vi "TagDB List Probe.vi"(11 "DB Ref":refnum<k1>) -> (2 "Value String":string, 3 "Boolean":bool)   [LabVIEW 2017]
uses:
  <vilib>/Utility/Data Type/Type Definitions/Data Type.ctl
  <vilib>/Utility/Data Type/Type Definitions/Refnum Type.ctl
  <vilib>/Utility/Data Type/Type Definitions/VI Server Generic Type.ctl
  TagDB/_Support/Change Detector/TagDB dbChanged.vi
  5c30c298-b379-4591-8ff9-b1fc8496978f.vi
  TagDB/_Support/DataAccess/TagDB Ref to DVR.vi
  TagDB/_Support/Error/_[error50000]Invalid DB REF.vi
  TagDB/_Support/Change Detector/TagDB ChangeFlag.vi
  TagDB/_Support/DataAccess/_NameCacher.vi
  TagDB/_Support/Error/_[error50002]Invalid DataType.vi
  TagDB/_Support/URL/TRIM-BOTH-SPACE.vi
  TagDB/_Support/Error/_Build Error Cluster.vi
  TagDB/TagDB.lvlib
  <vilib>/Utility/Data Type/NI_Data Type.lvlib
panel:
  out "Valid?":bool
  out "Name":string
  out "Last Item Change":timestamp format="%<%.3X>T"
  out "Last Data Change":timestamp format="%<%.3X>T"
  in  "Items":i32(listbox)
  out "TagName":string
  out "ValidRef":bool
  out "ClassName":string
  out "Type":T1
  out "Reference Type":T2
  out "VI Server Type":T3
  out "data":variant
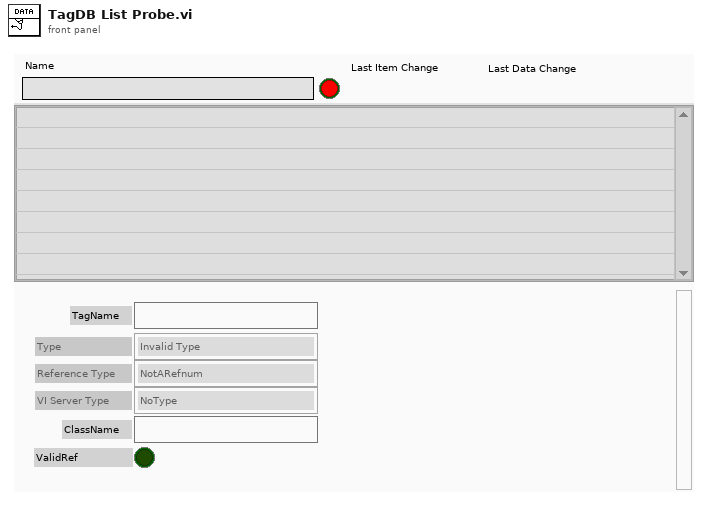
[diagram p1: front panel]
types:
  T1 = typedef "NI_Data Type.lvlib/Data Type.ctl" = enum8{"Invalid Type", "Void", "I8", "I16", "I32", "I64", "U8", "U16", "U32", "U64", "Single Float", "Double Float", "Extended Float", "Single Complex", "Double Complex", "Extended Complex", "Enum U8", "Enum U16", "Enum U32", "Enum U64", "Single Float With Unit", "Double Float With Unit", "Extended Float With Unit", "Single Complex with Unit", "Double Complex with Unit", "Extended Complex with Unit", "Boolean", "String", "Path", "Picture", "Tag", "Array", "Cluster", "Variant", "LV Variant", "Waveform", "Timestamp", "Digital Waveform", "Digital Data", "ExpressData", "Refnum", "External Data", "VI", "Poly VI", "LabVIEW Class Instance", "Fixed Point"}
  T2 = typedef "NI_Data Type.lvlib/Refnum Type.ctl" = enum16{"NotARefnum", "UnknownRefnum", "Generic", "Datalog", "ByteStream", "Device", "Occurence", "TCPNetConnection", "Auto", "Menu", "Imaq", "Hardware", "DataSocket", "Visa", "IVI", "UDPNetConnection", "Notifier", "Queue", "Irda", "EventReg", "DotNet", "UserEvent", "Callback", "UNUSED_EMPTY_POSITION", "BlueToothNetConnection", "LVObjApp", "LVObjVI", "LVObjUnknown", "GenericClass", "UserDefinedRefnumTag", "DataValue", "RT FIFO", "TDMS File"}
  T3 = typedef "NI_Data Type.lvlib/VI Server Generic Type.ctl" = enum16{"NoType", "\tkLVObjApp=0x1", "\tkLVObjVI", "\tkLVObjGeneric", "\tkLVObjDecoration", "\tkLVObjText", "\tkLVObjControl", "\tkLVObjColorBox", "\tkLVObjBoolean", "\tkLVObjRefNum", "\tkLVObjVariant", "\tkLVObjPath", "\tkLVObjListBox", "\tkLVObjTable", "\tkLVObjArray", "\tkLVObjPicture", "\tkLVObjOleContainer", "\tkLVObjNumeric", "\tkLVObjDigital", "\tkLVObjNamedNumeric", "\tkLVObjColorRamp", "\tkLVObjSlide", "\tkLVObjGraphOrChart", "\tkLVObjWaveformChart", "\tkLVObjWaveformGraph", "\tkLVObjIntensityChart", "\tkLVObjIntensityGraph", "\tkLVObjString", "\tkLVObjIOName", "\tkLVObjComboBox", "\tkLVObjCluster", "\tkLVObjPanel", "\tkLVObjKnob", "\tkLVObjNumWithScale", "\tkLVObjRing", "\tkLVObjEnum", "\tkLVObjGObject", "\tkLVObjPlot", "\tkLVObjCursor", "\tkLVObjNumericText", "\tkLVObjScale", "\tkLVObjColorScale", "\tkLVObjGraphScale", "\tkLVObjColorGraphScale", "\tkLVObjTypedRefNum", "\tkLVObjOldKnobScale", "\tkLVObjMCListbox", "\tkLVObjMeasureData", "\tkLVObjDSCTag", "\tkLVObjDAQName", "\tkLVObjVISAName", "\tkLVObjIVIName", "\tkLVObjSlideScale", "\tkLVObjTabControl", "\tkLVObjPage", "\tkLVObjTabArrayTabControl", "\tkLVObjConPane", "\tkLVObjDAQMXName", "\tkLVObjVIRefNum", "\tkLVObjLVObjRefNum", "\tkLVObjAbsTime", "\tkLVObjDigitalTable", "\tkLVObjUnused", "\tkLVObjUnused2", "\tkLVObjSCLControl", "\tkLVObjSubPanel", "\tkLVObjTreeControl", "\tkLVObjGenClassTagRef", "\tkLVObjGenClassRef", "\tkLVObjRotaryColorScale", "\tkLVObjPlugInDDOControl", "\tkLVObjPlugInDDOClassHolder", "\tkLVObjRadClusControl", "\tkLVObjProject", "\tkLVObjProjectItem", "\tkLVObjPane", "\tkLVObjSplitterBar", "\tkLVObjProjectBuildItem", "\tkLVObjPixmap", "\tkLVObjFacadeVI", "\tkLVObjLibrary", "\tkLVObjVariable", "\tkLVObjPropertyBag", "\tkLVObjXYGraph", "\tkLVObjScene", "\tkLVObjUDClassLibrary", "\tkLVObjUDClassClone", "\tkLVObjMethodVI", "\tkLVObjXCtlLibrary", "\tkLVObjXNodeLibrary", "\tkLVObjScroll", "\tkLVObjLVTarget", "\tkLVObjMixedGraph", "\tkLVObjProvider", "\tkLVObjCopyOperation", "\tkLVObjTargetItem", "\tkLVObjProjectItemType", "\tkLVObjCopyItem", "\tkLVObjCopyConflict", "\tkLVObjCopyExpert", "\tkLVObjSceneGraphDisp", "\tkLVObjPolyVI", "\tkLVObjLVClassDDO", "kLVObjDiagram=0x4000", "\tkLVObjTerminal", "\tkLVObjConstant", "\tkLVObjPathConstant", "\tkLVObjArrayConstant", "\tkLVObjNumericConstant", "\tkLVObjDigitalNumConstant", "\tkLVObjNamedNumericConstant", "\tkLVObjStringConstant", "\tkLVObjClusterConstant", "\tkLVObjFixedConstant", "\tkLVObjControlTerminal", "\tkLVObjFormulaParameter", "\tkLVObjGlobal", "\tkLVObjLocal", "\tkLVObjRightShiftRegister", "\tkLVObjFunction", "\tkLVObjSubVI", "\tkLVObjCallByRef", "\tkLVObjUnitCast", "\tkLVObjStructure", "\tkLVObjLoop", "\tkLVObjMultiframeStructure", "\tkLVObjSequence", "\tkLVObjCaseSelector", "\tkLVObjFormula", "\tkLVObjGrowableFunction", "\tkLVObjBuildClusterArray", "\tkLVObjCompoundArithmetic", "\tkLVObjIndexArray", "\tkLVObjBuildArray", "\tkLVObjNamedBundler", "\tkLVObjCIN", "\tkLVObjCallLibrary", "\tkLVObjObjectFunction", "\tkLVObjProperty", "\tkLVObjInvoke", "\tkLVObjNode", "\tkLVObjBooleanConstant", "\tkLVObjBlockDiagram", "\tkLVObjRingConstant", "\tkLVObjEnumConstant", "\tkLVObjTunnel", "\tkLVObjLoopTunnel", "\tkLVObjSequenceLocal", "\tkLVObjComparison", "\tkLVObjReadWriteFile", "\tkLVObjTypeCast", "\tkLVObjFlattenUnflattenString", "\tkLVObjGPIBReadWrite", "\tkLVObjForLoop", "\tkLVObjWhileLoop", "\tkLVObjScriptNode", "\tkLVObjArrayToCluster", "\tkLVObjFormatScanString", "\tkLVObjWire", "\tkLVObjProbe", "\tkLVObjInnerTerminal", "\tkLVObjLeftShiftRegister", "\tkLVObjPolySubVI", "\tkLVObjPropItem", "\tkLVObjIONameConstant", "\tkLVObjDSCTagConstant", "\tkLVObjDAQNameConstant", "\tkLVObjVISANameConstant", "\tkLVObjIVINameConstant", "\tkLVObjColorBoxConstant", "\tkLVObjControlRefConstant", "\tkLVObjClassSpecifierConstant", "\tkLVObjConfNode", "\tkLVObjMasterWizard", "\tkLVObjStateDiagWizard", "\tkLVObjOuterTerminal", "\tkLVObjDAQMXNameConstant", "\tkLVObjEventStructure", "\tkLVObjFlatSequence", "\tkLVObjGenClassTagRefConstant", "\tkLVObjAbsTimeConstant", "\tkLVObjExternalNode", "\tkLVObjSubWizard", "\tkLVObjScriptNodeParameter", "\tkLVObjStatVIRef", "\tkLVObjComboBoxConstant", "\tkLVObjTimedLoop", "\tkLVObjGenClassDeepCopy", "\tkLVObjGenClassTagFlat", "\tkLVObjGenClassTagFlatRefConstant", "\tkLVObjGenClassFlat", "\tkLVObjSimDiagram", "\tkLVObjCompDiagram", "\tkLVObjSimNode", "\tkLVObjSimDCO", "\tkLVObjBundler", "\tkLVObjUnbundler", "\tkLVObjNamedUnbundler", "\tkLVObjFlatSeqFrame", "\tkLVObjFlatSeqInTun", "\tkLVObjFlatSeqOutTun", "\tkLVObjRefNumConst", "\tkLVObjFlattenString", "\tkLVObjPolySelector", "\tkLVObjXNode", "\tkLVObjSelectorTunnel", "\tkLVObjCommentNode", "\tkLVObjSdfDiagram", "\tkLVObjSDFCompDiagram", "\tkLVObjSdfNode", "\tkLVObjSdfDCO", "\tkLVObjFileDialog", "\tkLVObjTLDCO", "\tkLVObjTimeSeqFrame", "\tkLVObjTimeFlatSequence", "\tkLVObjTimedSequence", "\tkLVObjXDataNode", "\tkLVObjCodeWizard", "\tkLVObjMathScriptNode", "\tkLVObjMathScriptNodeParameter", "\tkLVObjLVClassBDConst"}
  T4 = enum8{"Enabled", "Disabled", "Disabled and Grayed Out"}
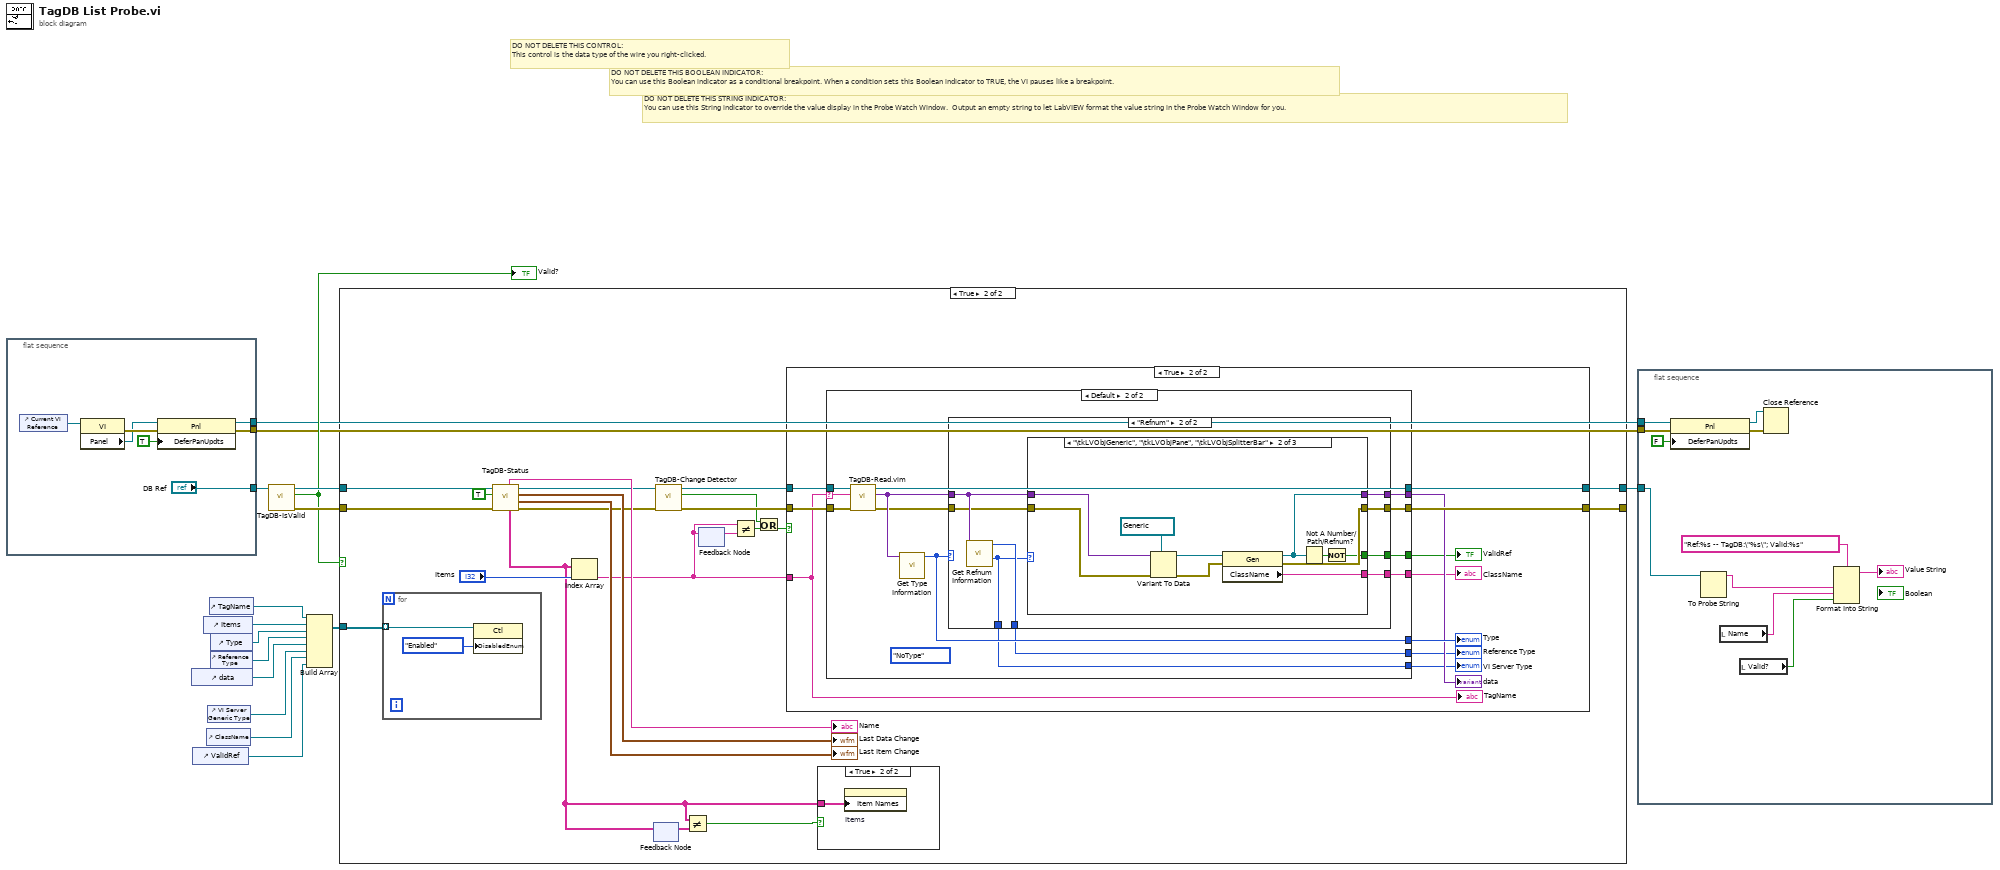
[diagram p0: block diagram]
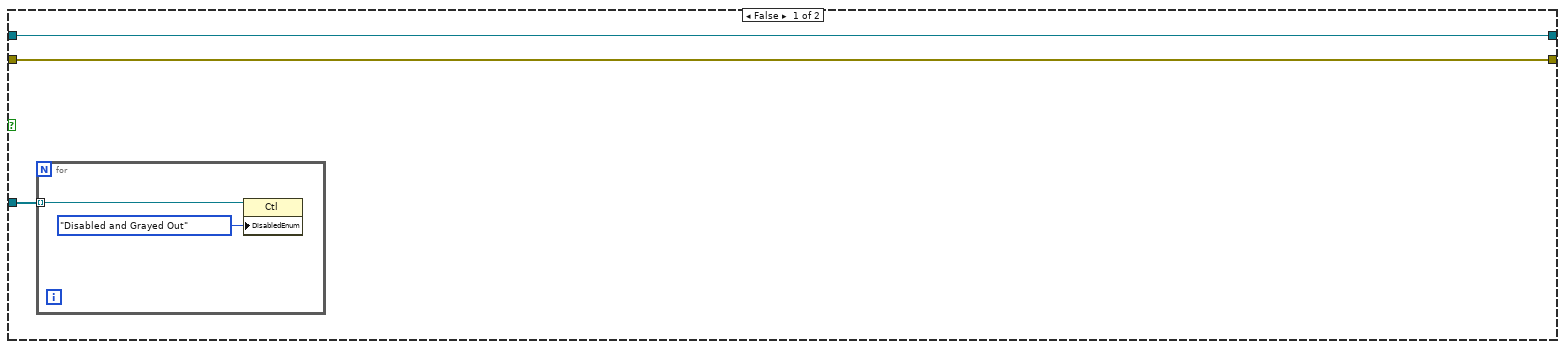
[diagram p2: hidden frame]
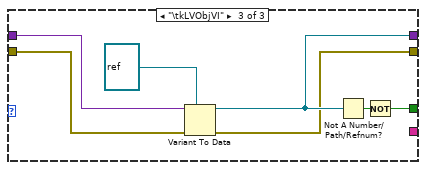
[diagram p7: hidden frame]
diagram:
  # "DO NOT DELETE THIS STRING INDICATOR: \nYou can use this String indicator to override the value display in the Probe Watch Window.  Output an empty string to let LabVIEW format the value string in the Probe Watch Window for you."
  # "DO NOT DELETE THIS BOOLEAN INDICATOR: \nYou can use this Boolean indicator as a conditional breakpoint. When a condition sets this Boolean indicator to TRUE, the VI pauses like a breakpoint."
  # "DO NOT DELETE THIS CONTROL: \nThis control is the data type of the wire you right-clicked."
  n1 = flat-sequence {
    tunnel: ["DB Ref"] -> w14
    tunnel: [w18] -> w6
    tunnel: [w17] -> w5
    frame #0 {
      n2 = control-ref of="Current VI Reference"() -> (w22:refnum<vi>)
      n3 = property class="VI"(reference=w22) -> (error out=w21:errorcluster, "Panel"=w20:refnum<vi>)  [unwired: 1 in, 1 out]
      n4 = property class="Pnl"(reference=w20, error in=w21, "DeferPanUpdts"=TRUE ("Defer Panel Updates")) -> (reference out=w18:refnum<vi>, error out=w17:errorcluster)
    }
  }
  n5 = control-ref of="data"() -> (w9:refnum<vi>)
  n6 = control-ref of="ValidRef"() -> (w2:refnum<vi>)
  n7 = control-ref of="Items"() -> (w12:refnum<vi>)
  n8 = control-ref of="ClassName"() -> (w3:refnum<vi>)
  n9 = control-ref of="VI Server Generic Type"() -> (w4:refnum<vi>)
  n10 = control-ref of="TagName"() -> (w1:refnum<vi>)
  n11 = control-ref of="Type"() -> (w11:refnum<vi>)
  n12 = control-ref of="Reference Type"() -> (w10:refnum<vi>)
  n13 = call "TagDB-IsValid.vi"("TagDB"=w14) -> ("error out"=w15:errorcluster, "valid TagDB?"=w13:bool, "TagDB(dup)"=w16:refnum<k1>)  [unwired: 8 in]
  "Valid?" <- w13
  n14 = Build Array(w1, w12, w11, w10, w9, w4, w3, w2) -> (w8:refnum<vi>[])
  n15 = case shown="True" w13 {
    tunnel: w16 -> [w25 w50]
    tunnel: w15 -> [w24 w49]
    tunnel: w8 -> [w26 w43]
    tunnel: [w25 w42] -> w7
    tunnel: [w24 w41] -> _
    frame False {
      n16 = for {
        tunnel: w26 -> [w27] mode=indexing
        n17 = property class="Ctl"(reference=w27, "DisabledEnum"=T4."Disabled and Grayed Out" ("Disabled")) -> ()  [unwired: 1 in, 2 out]
      }
    }
    frame True {
      n18 = for {
        tunnel: w43 -> [w109] mode=indexing
        n19 = property class="Ctl"(reference=w109, "DisabledEnum"=T4."Enabled" ("Disabled")) -> ()  [unwired: 1 in, 2 out]
      }
      n20 = call "TagDB-Status.vi"("error in (no error)"=w49, "return elements? (F)"=TRUE, "DB Ref"=w50) -> ("error out"=w35:errorcluster, "Item Change Timestamp"=→"Last Item Change":timestamp, "Global Change Timestamp"=→"Last Data Change":timestamp, "DB Ref(dup)"=w44:refnum<k1>, "DB items"=w38:string[], "db name"=→"Name":string)  [unwired: 3 in]
      n21 = Index Array(array=w38, index="Items") -> (element=w32:string)
      n22 = feedback-in #1(w38) -> ()
      n23 = feedback #1() -> (w39:string[])  [unwired: 1 in]
      n24 = call-poly "TagDB-Change Detector.vi"("error in (no error)"=w35, "DB Ref"=w44) -> ("error in (no error) (dup)"=w34:errorcluster, "changed?"=w29:bool, "DB Ref (dup)"=w36:refnum<k1>)  [unwired: 7 in]
      n25 = Not Equal?(x=w38, y=w39) -> (x != y?=w37:bool)
      n26 = feedback #2() -> (w33:string)  [unwired: 1 in]
      n27 = feedback-in #2(w32) -> ()
      n28 = Not Equal?(x=w32, y=w33) -> (x != y?=w31:bool)
      n29 = Or(x=w29, y=w31) -> (x .or. y?=w30:bool)
      n30 = case shown="True" w30 {
        tunnel: [w52 w63] -> w42
        tunnel: [w51 w62] -> w41
        tunnel: w36 -> [w52 w57]
        tunnel: w34 -> [w51 w56]
        tunnel: w32 -> [_ w53]
        frame False {
        }
        frame True {
          n31 = case shown="Default" w53 {
            selector: w53 -> [_ w77]
            tunnel: w57 -> [w65 w78]
            tunnel: [w65 w76] -> w63
            tunnel: [w64 w71] -> w62
            tunnel: [_ w74] -> w60
            tunnel: w56 -> [w64 w75]
            tunnel: [_ w70] -> w61
            tunnel: [_ w69] -> w59
            tunnel: [_ w68] -> w58
            tunnel: [_ w67] -> w55
            tunnel: [_ w66] -> w54
            frame "" {
            }
            frame Default {
              (unwired) VI_Server_Generic_Type."NoType" ("VI Server Generic Type")
              n32 = call "TagDB-Read.vim"("error in (no error)"=w75, "name"=w77, "TagDB"=w78) -> ("error out"=w72:errorcluster, "Value"=w73:variant, "TagDB(dup)"=w76:refnum<k1>)  [unwired: 3 in, 3 out]
              n33 = call <vilib>:"Get Type Information.vi"("Variant"=w73) -> ("Type"=w70:T1)  [unwired: 6 in, 4 out]
              n34 = case shown="\"Refnum\"" w70 {
                tunnel: [w80 w88] -> w74
                tunnel: w73 -> [w80 w87]
                tunnel: w72 -> [w79 w86]
                tunnel: [w79 w85] -> w71
                tunnel: [_ w84] -> w69
                tunnel: [_ w81] -> w68
                tunnel: [_ w83] -> w67
                tunnel: [_ w82] -> w66
                frame Default {
                }
                frame "Refnum" {
                  n35 = call <vilib>:"Get Refnum Information.vi"("Variant"=w87) -> ("VI Server Generic Type"=w81:T3, "Reference Type"=w84:T2)  [unwired: 7 in, 2 out]
                  n36 = case shown="\"\\tkLVObjGeneric\", \"\\tkLVObjPane\", \"\\tkLVObjSplitterBar\"" w81 {
                    tunnel: [w89 w92 w106] -> w88
                    tunnel: w87 -> [w89 w100 w107]
                    tunnel: w86 -> [w90 w97 w105]
                    tunnel: [w90 w96 w104] -> w85
                    tunnel: [_ w95 _] -> w83
                    tunnel: [_ w93 w102] -> w82
                    frame Default {
                    }
                    frame "\tkLVObjGeneric", "\tkLVObjPane", "\tkLVObjSplitterBar" {
                      n37 = Variant To Data(error in=w97, type=refnum<vi> refnum ("value"), Variant=w100) -> (data=w98:refnum<vi>, error out=w91:errorcluster)
                      n38 = property class="Gen"(reference=w98, error in=w91) -> (reference out=w92:refnum<vi>, error out=w96:errorcluster, "ClassName"=w95:string)
                      n39 = Not A Number/Path/Refnum?(number/path/refnum=w92) -> (NaN/Path/Refnum?=w94:bool)
                      n40 = Not(x=w94) -> (.not. x?=w93:bool)
                    }
                    frame "\tkLVObjVI" {
                      n41 = Variant To Data(error in=w105, type=refnum<vi> refnum ("Current VI Reference"), Variant=w107) -> (data=w106:refnum<vi>, error out=w104:errorcluster)
                      n42 = Not A Number/Path/Refnum?(number/path/refnum=w106) -> (NaN/Path/Refnum?=w103:bool)
                      n43 = Not(x=w103) -> (.not. x?=w102:bool)
                    }
                  }
                }
              }
            }
          }
          "data" <- w60
          "Type" <- w61
          "Reference Type" <- w59
          "VI Server Type" <- w58
          "ClassName" <- w55
          "ValidRef" <- w54
          "TagName" <- w53
        }
      }
      n44 = case shown="True" w37 {
        tunnel: w38 -> [_ w108]
        frame False {
        }
        frame True {
          n45 = property on="Items" class="LstBox (strict)"("Item Names"=w108) -> ()  [unwired: 2 in, 2 out]
        }
      }
    }
  }
  n46 = flat-sequence {
    tunnel: w7 -> [w115]
    tunnel: w6 -> [w120]
    tunnel: w5 -> [w119]
    frame #0 {
      n47 = property class="Pnl"(reference=w120, error in=w119, "DeferPanUpdts"=FALSE ("Defer Panel Updates")) -> (reference out=w117:refnum<vi>, error out=w118:errorcluster)
      n48 = To Probe String(7:w115) -> (3:w114:string)  [unwired: 2 in, 1 out]
      n49 = local read "Name"() -> (w112:string)
      n50 = local read "Valid?"() -> (w113:bool)
      n51 = Close Reference(reference=w117, error in (no error)=w118) -> ()  [unwired: 1 out]
      n52 = Format Into String(format string="Ref:%s -- TagDB:\"%s\"; Valid:%s", w114, w112, w113) -> (resulting string=→"Value String":string)  [unwired: 2 in, 1 out]
    }
  }
